vi "Temperature_Calculation.vi"(10 "R":dbl, 11 "temp selection":string) -> (3 "temp":dbl)   [LabVIEW 2021]
panel:
  out "B value":dbl
  in  "To":dbl=298.15
  in  "Ro":dbl=10.0
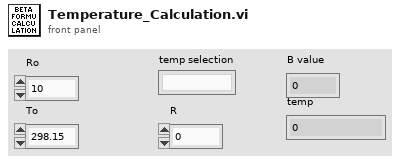
[diagram p1: front panel]
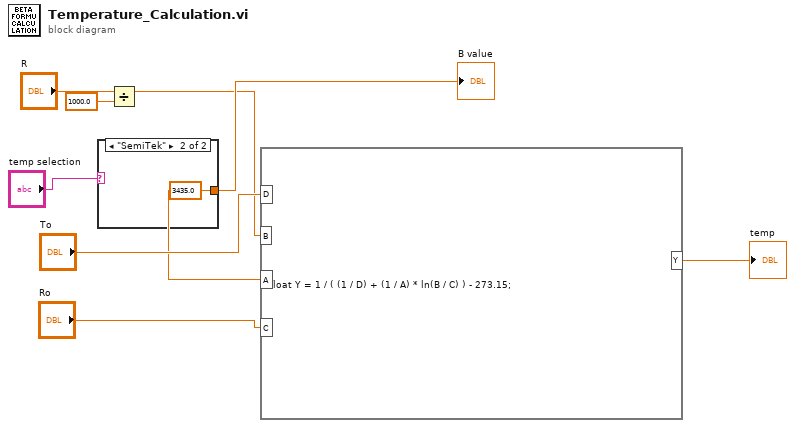
[diagram p0: block diagram]
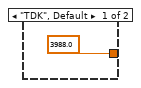
[diagram p2: hidden frame]
diagram:
  n1 = case shown="\"SemiTek\"" "temp selection" {
    tunnel: [3988.0 3435.0] -> w3
    frame "TDK", Default {
    }
    frame "SemiTek" {
    }
  }
  "B value" <- w3
  n2 = Divide(x="R", y=1000.0) -> (x/y=w2:dbl)
  n3 = formula code="float Y = 1 / ( (1 / D) + (1 / A) * ln(B / C) ) - 273.15;"("D"="To", "B"=w2, "A"=w3, "C"="Ro") -> ("Y"=→"temp":dbl)
